vi "WaitForCommand.vi"(8 "error in (no error)":errorcluster, 11 "ServiceManager-Comms in":refnum<class "ServiceManager-Comms.lvclass">) -> (0 "error out":errorcluster, 3 "ServiceManager-Comms out":refnum<class "ServiceManager-Comms.lvclass">)   [LabVIEW 2020, in "ServiceManager-Comms.lvlib" / "ServiceManager-Comms.lvclass"]
uses:
  ServiceManager-Comms.lvclass
  C:/Program Files (x86)/National Instruments/LabVIEW 2020/vi.lib/ActorFramework/Actor/Actor.lvclass
  ServiceManager-Comms Messages/WaitForCommand Msg/WaitForCommand Msg.lvclass
  C:/Program Files (x86)/National Instruments/LabVIEW 2020/vi.lib/ActorFramework/Message/Message.lvclass
  <vilib>/ActorFramework/Actor/Actor.lvclass
  ServiceManager Messages/Launch Downstream Handler Msg/Launch Downstream Handler Msg.lvclass
  C:/Users/taylo/Projects/g-go-service-fwrk/scratchpad/ServiceManagerBeta/ServiceManager/Nested/ServiceManager-Comms/ServiceManager-Comms.lvclass
  C:/Users/taylo/Projects/g-go-service-fwrk/scratchpad/ServiceManagerBeta/ServiceManager/Message Handling/Message Handling.lvclass
  C:/Users/taylo/Projects/g-go-service-fwrk/scratchpad/ServiceManagerBeta/ServiceManager/Nested/ServiceManager-Comms/ServiceManager-Comms Messages/WaitForCommand Msg/WaitForCommand Msg.lvclass
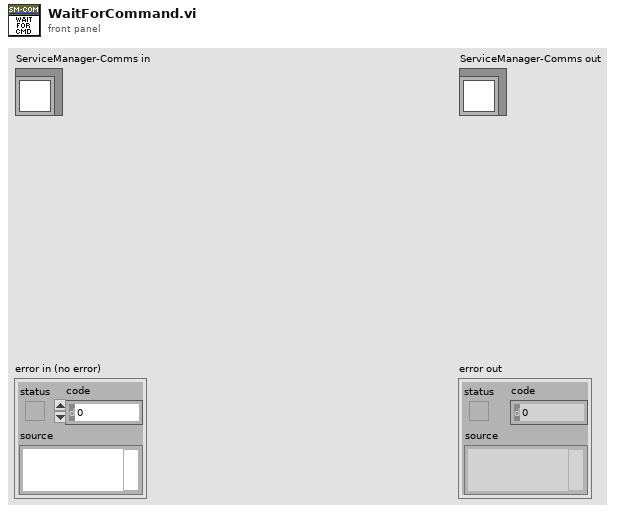
[diagram p1: front panel]
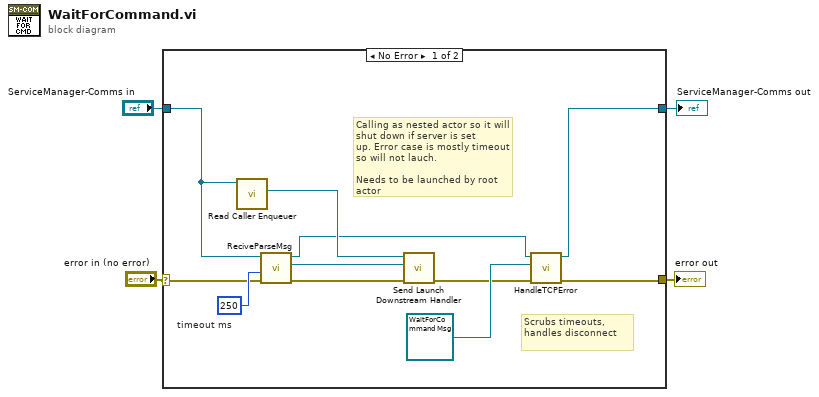
[diagram p0: block diagram]
diagram:
  n1 = case shown="No Error" "error in (no error)" {
    selector: "error in (no error)" -> [w14 w17]
    tunnel: [w11 w17] -> w3
    tunnel: [w12 w16] -> w1
    tunnel: "ServiceManager-Comms in" -> [w10 w16]
    frame No Error {
      w15 = 250  # timeout ms
      # "Scrubs timeouts, handles disconnect"
      # "Calling as nested actor so it will shut down if server is set \nup. Error case is mostly timeout so will not lauch.\n\nNeeds to be launched by root actor"
      n2 = call <vilib>:"Read Caller Enqueuer.vi"("Actor"=w10) -> ("Caller Enqueuer"=w9:refnum<class "Message Enqueuer.lvclass">)  [unwired: 10 in]
      n3 = call-dynamic "ReciveParseMsg.vi"("error in (no error)"=w14, "timeout ms (25000)"=w15, "ServiceManager-Comms in"=w10) -> ("error out"=w8:errorcluster, "DownStreamMsgHandler"=w5:refnum<class "DownStreamMsgHandler.lvclass">, "ServiceManager-Comms out"=w7:refnum<class "ServiceManager-Comms.lvclass">)  [unwired: 6 in]
      n4 = call "Send Launch Downstream Handler.vi"("error in (no error)"=w8, "DownStreamMsgHandler"=w5, "Message Enqueuer"=w9) -> ("error out"=w6:errorcluster)  [unwired: 7 in, 1 out]
      n5 = call "HandleTCPError.vi"("error in (no error)"=w6, "NoErrorMessage"=refnum<class "WaitForCommand Msg.lvclass"> refnum ("ServiceManager.lvlib:WaitForCommand Msg.lvclass"), "ServiceManager-Comms in"=w7) -> ("error out"=w11:errorcluster, "ServiceManager-Comms out"=w12:refnum<class "ServiceManager-Comms.lvclass">)  [unwired: 7 in]
    }
    frame Error {
    }
  }
  "error out" <- w3
  "ServiceManager-Comms out" <- w1
